vi "读取选择目录.vi"(8 "error in (no error)":errorcluster caption="错误输入（无错误）", 11 "奶茶输入":refnum<class "奶茶.lvclass">) -> (0 "error out":errorcluster caption="错误输出", 2 "选择目录":u16(ring) items=["黑糯米奶茶", "招牌奶茶", "茉莉奶茶"], 3 "奶茶输出":refnum<class "奶茶.lvclass">)   [LabVIEW 2016, in "奶茶.lvclass"]
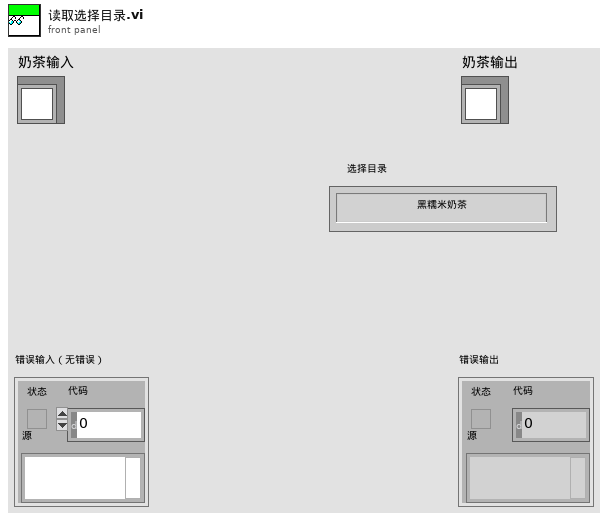
[diagram p1: front panel]
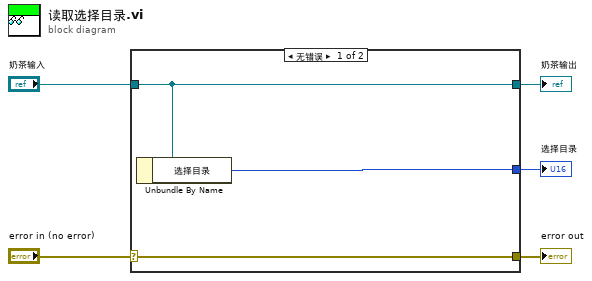
[diagram p0: block diagram]
diagram:
  n1 = case shown="无错误" "error in (no error)" {
    selector: "error in (no error)" -> [w8 w9]
    tunnel: [w8 w9] -> w4
    tunnel: [w7 w10] -> w2
    tunnel: "奶茶输入" -> [w7 w10]
    tunnel: [w6 _] -> w1
    frame No Error {
      n2 = Unbundle By Name(w7) -> ("选择目录"=w6:u16)
    }
    frame Error {
    }
  }
  "error out" <- w4
  "奶茶输出" <- w2
  "选择目录" <- w1
